vi "Close Log File.vi"(8 "error in (no error)":errorcluster, 11 "tdms file":refnum<k34>) -> (0 "error out":errorcluster)   [LabVIEW 2017, in "Logging.lvlib"]
uses:
  Logging.lvlib
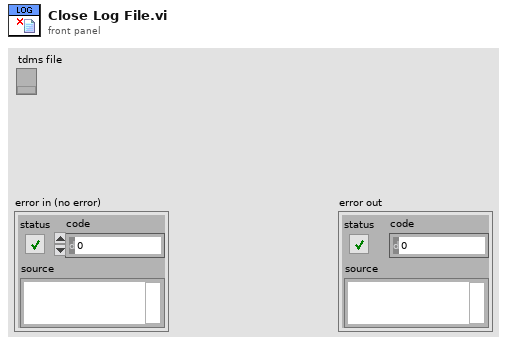
[diagram p1: front panel]
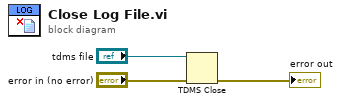
[diagram p0: block diagram]
diagram:
  n1 = TDMS Close(8:"error in (no error)", 11:"tdms file") -> (0:→"error out":errorcluster)  [unwired: 1 out]
